vi "WCL.vi"(0 "System no.":i32=1 min=1 max=4 step=1, 2 "WCL axes":string[](array[string]), 3 "All axes?":bool, 4 "Axis identifier?":bool=TRUE, 5 "error in":errorcluster) -> (19 "error out":errorcluster)   [LabVIEW 2026]
doc: "Clears waveform associated with specified axis.\n\nC-413: WCL axes is identical with wave table number which can be 1 to 8. All axes? must be FALSE. \n\nC-886: WCL axes is identical with wave table number which can be 1 to 100. All axes? must be FALSE.\n\nC-887: WCL axes is identical with wave table number which can be 1 to 100. All axes? must be FALSE.\n\nE-517, E-518: WCL axes is identical with wave table number which can be 1 to 3. All axes? must be FALSE.\n\nE-709: WCL axes is identical with wave table number which can be 1 to 6. All axes? must be FALSE. \n\nE-710: Does also clear DDL table. All axes must be FALSE, only one axis per command allowed. \n\nE-712: WCL axes is identical with wave table number which can be 1 to 90. All axes? must be FALSE. \n\nE-725: WCL axes is identical with wave table number which can be 1 to 30. All axes? must be FALSE. \n\nE-727: WCL axes is identical with wave table number which can be 1 to 40. All axes? must be FALSE. \n\nE-753: WCL axes is identical with wave table number which can be 1 to 10. All axes? must be FALSE. \n\nE-754: WCL axes is identical with wave table number which can be 1 to 10. All axes? must be FALSE. \n\nE-761: All axes must be FALSE."
panel:
  # "Clears waveform associated with specified axis."
  # "If all axes: use"
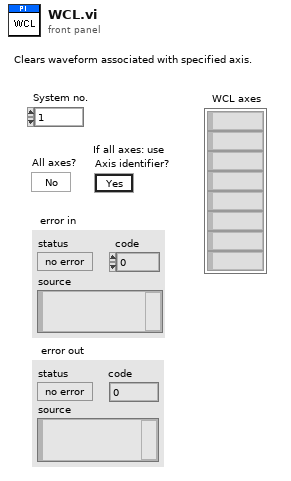
[diagram p1: front panel]
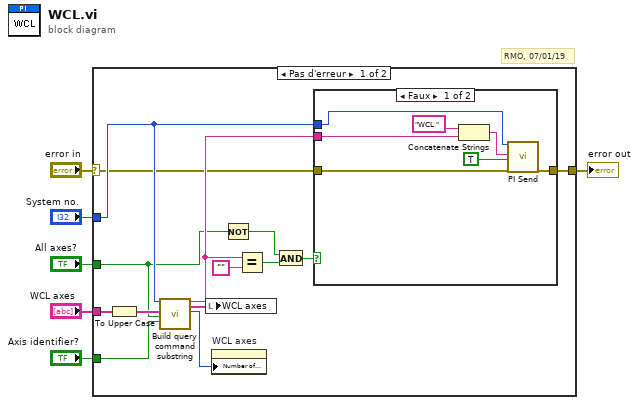
[diagram p0: block diagram]
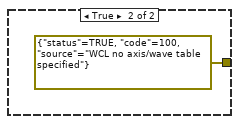
[diagram p2: hidden frame]
diagram:
  # "RMO, 07/01/19"
  n1 = case shown="Pas d'erreur" "error in" {
    selector: "error in" -> [w9 w29]
    tunnel: "WCL axes" -> [w20 _]
    tunnel: "Axis identifier?" -> [w17 _]
    tunnel: "System no." -> [w15 _]
    tunnel: "All axes?" -> [w11 _]
    tunnel: [w8 w29] -> w2
    frame No Error {
      n2 = To Upper Case(1:w20) -> (0:w18:string[])
      n3 = call "Build query command substring.vi"("System no."=w15, "Axes to query in"=w18, "Query\nAll axes?"=w11, "For all axes: use\nAxis identifier?"=w17) -> ("Command substring"=w16:string, "Axes to query out"=w14:string[], "Number of rows"=w13:u32)  [unwired: 2 in, 11 out]
      n4 = local write "WCL axes"(w14) -> ()
      n5 = property on="WCL axes" class="Tabl (strict)"("Number of Rows"=w13) -> ()  [unwired: 2 in, 2 out]
      n6 = Not(x=w11) -> (.not. x?=w10:bool)
      n7 = Equal?(x=w16, y="" ("x")) -> (x = y?=w12:bool)
      n8 = And(x=w10, y=w12) -> (x .and. y?=w7:bool)
      n9 = case shown="Faux" w7 {
        tunnel: w16 -> [w24 _]
        tunnel: w15 -> [w23 _]
        tunnel: w9 -> [w22 _]
        tunnel: [w21 errorcluster {"status"=TRUE, "code"=100, "source"="WCL no axis/wave table specified"} ("error out")] -> w8
        frame False {
          n10 = Concatenate Strings("WCL ", w24) -> (w25:string)
          n11 = call "PI Send.vi"("System no."=w23, "String to send"=w25, "Attach termination char.?"=TRUE ("Attach Linefeed?"), "error in"=w22) -> ("error out"=w21:errorcluster)  [unwired: 2 in, 13 out]
        }
        frame True {
        }
      }
    }
    frame Error {
    }
  }
  "error out" <- w2
